vi "Save PNG Image (Path).vi"(8 "error in (no error)":errorcluster, 9 "Compression (6)":i32=6, 10 "Image":T1, 11 "Path In":path) -> (0 "error out":errorcluster, 3 "Path Out":path)   [LabVIEW 2020, in "G-Image.lvlib"]
doc: "Saves an image in PNG format to disk.\n\nThe <b>Compression</b> input sets the compression level of the PNG image., ranging from 0 (no compression) to 10 (maximum compression). Values outside this range will be coerced in range."
uses:
  G-Image.lvlib
  <vilib>/picture/picture.llb/imagedata.ctl
  Controls/Image Save Format.ctl
  ec7aa72e-e6e2-44af-9f17-7fe58dd5f276.vi
  Private/Result To Error.vi
  Private/Get Image Data.vi
  Private/ARGB To RGBA.vi
  Private/Depth To Number Channels.vi
  Image Processing/Indexed Color To True Color Image.vi
  <vilib>/Utility/error.llb/Error Cluster From Error Code.vi
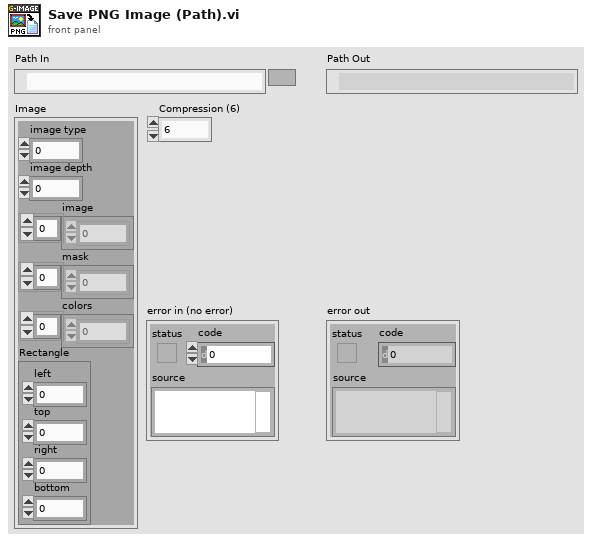
[diagram p1: front panel]
types:
  T1 = typedef "imagedata.ctl" = cluster{"image type":i32, "image depth":i32, "image":u8[], "mask":u8[], "colors":u32[], "Rectangle":cluster{"left":i16, "top":i16, "right":i16, "bottom":i16}}
  T2 = typedef "G-Image.lvlib/Image Save Format.ctl" = enum16{"png", "jpg", "bmp", "gif", "tga"}
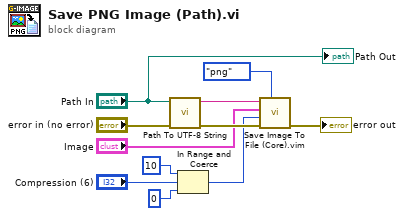
[diagram p0: block diagram]
diagram:
  n1 = call "Path To UTF-8 String.vi"("error in"="error in (no error)", "Path"="Path In") -> ("error out"=w7:errorcluster, "UTF-8 String"=w10:string)  [unwired: 8 in]
  n2 = In Range and Coerce(upper limit=10, x="Compression (6)", lower limit=0) -> (coerced(x)=w3:i32)  [unwired: 1 out]
  n3 = call "Save Image To File (Core).vim"("Save Format"=Image_Save_Format."png", "error in (no error)"=w7, "Option"=w3, "Picture"="Image", "Path In"=w10) -> ("error out"=→"error out":errorcluster)  [unwired: 5 in, 1 out]
  "Path Out" <- "Path In"
